vi "Merge Directories.vi"(6 "Ignore Read-Only? (FALSE)":bool, 8 "error in (no error)":errorcluster, 9 "Overwrite Existing Files? (FALSE)":bool, 10 "target directory path":path, 11 "source directory path":path) -> (0 "error out":errorcluster, 3 "dup target directory path":path)   [LabVIEW 2024]
doc: "Copies the contents of source directory into the destination directory. If source directory has subdirectories they will be copied into the destination directory recursively. Optionally, existing files may be overwritten, by setting the \"Overwrite Existing Files?\" input to TRUE. If you attempt to overwrite an existing file without setting to TRUE ans error will be returned. If FALSE, existing files will not be overwritten and no error wil be returned, Optionally, read-only files may be overwritten, by setting the \"Ignore Read-Only?\" input to TRUE. If you attempt to overwrite a read-only files without setting to TRUE an error will be returned. Optionally, by setting the \"Delete Source?\" input to TRUE the source directory will be deleted upon merge completion if no errors occured."
uses:
  <userlib>/_OpenG.lib/file/file.llb/Build Path - File Names Array__ogtk.vi
  <userlib>/_OpenG.lib/file/file.llb/Compare Two Paths - Scalar__ogtk.vi
  <userlib>/_OpenG.lib/file/file.llb/Build Path - Traditional - path__ogtk.vi
  <userlib>/_OpenG.lib/file/file.llb/Strip Path - Traditional__ogtk.vi
  <userlib>/_OpenG.lib/file/file.llb/openg_file.lvlib
  <userlib>/_OpenG.lib/error/error.llb/openg_error.lvlib
panel:
  # "OpenG Library.vi\n\nMerge Directories.vi\n\nCopies the contents of source directory into the destination directory.\n\nPlease visit http://www.OpenG.org to learn about the\nOpen Source LabVIEW software movement.\n\nNOTICE -- YOU MUST LEAVE THIS NOTICE IN PLACE.  PER THE TERMS OF THE LICENSE BELOW, YOU MAY SUBLICENSE THIS SOFTWARE \nIN ANY WAY THAT DOES NOT CONFLICT WITH THIS LICENSE.\n\n### BSD License (http://www.opensource.org/licenses/bsd-license.php) Begin ###\n \nCopyright (c) 2002-2004, Jim Kring <jim@jimkring.com>\nCopyright (c) 2002, Cal-Bay Systems, Inc. <info@calbay.com>\n\nAll rights reserved.\n\nRedistribution and use in source and binary forms, with or without modification, are permitted provided that the following conditions are met:\n\n    * Redistributions of source code must retain the above copyright notice, this list of conditions and the following disclaimer.\n    * Redistributions in binary form must reproduce the above copyright notice, this list of conditions and the following disclaimer in the \n       documentation and/or other materials provided with the distribution.\n    * Neither the name of SciWare, James Kring, Inc., nor the names of its contributors may be used to endorse or promote products derived \n       from this software without specific prior written permission.\n\nTHIS SOFTWARE IS PROVIDED BY THE COPYRIGHT HOLDERS AND CONTRIBUTORS \"AS IS\" AND ANY EXPRESS OR IMPLIED WARRANTIES, \nINCLUDING, BUT NOT LIMITED TO, THE IMPLIED WARRANTIES OF MERCHANTABILITY AND FITNESS FOR A PARTICULAR PURPOSE ARE \nDISCLAIMED. IN NO EVENT SHALL THE COPYRIGHT OWNER OR CONTRIBUTORS BE LIABLE FOR ANY DIRECT, INDIRECT, INCIDENTAL,\n SPECIAL, EXEMPLARY, OR CONSEQUENTIAL DAMAGES (INCLUDING, BUT NOT LIMITED TO, PROCUREMENT OF SUBSTITUTE GOODS OR \nSERVICES; LOSS OF USE, DATA, OR PROFITS; OR BUSINESS INTERRUPTION) HOWEVER CAUSED AND ON ANY THEORY OF LIABILITY, \nWHETHER IN CONTRACT, STRICT LIABILITY, OR TORT (INCLUDING NEGLIGENCE OR OTHERWISE) ARISING IN ANY WAY OUT OF THE USE \nOF THIS SOFTWARE, EVEN IF ADVISED OF THE POSSIBILITY OF SUCH DAMAGE.\n\n### BSD License End ###"
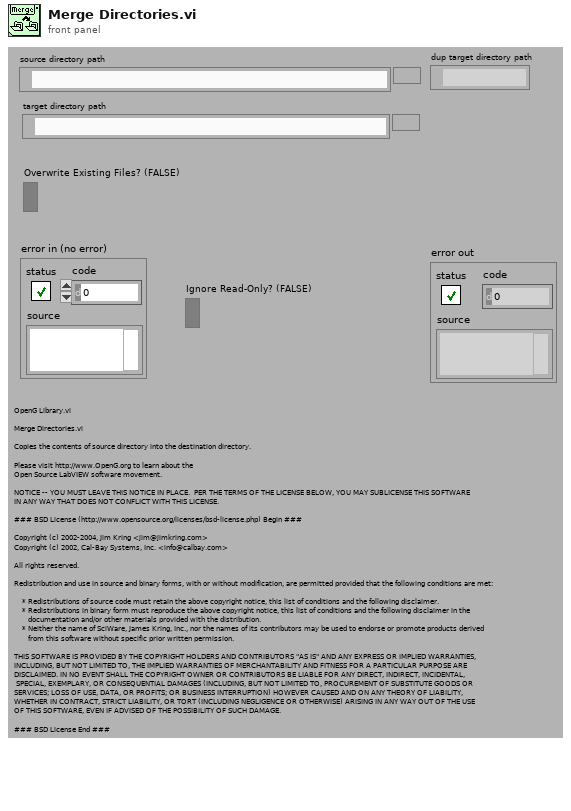
[diagram p1: front panel]
types:
  T1 = cluster{"Archive":bool, "Normal":bool, "Temporary":bool, "Compressed":bool, "Offline":bool, "Content Indexed":bool, "Encrypted (cannot set)":bool}
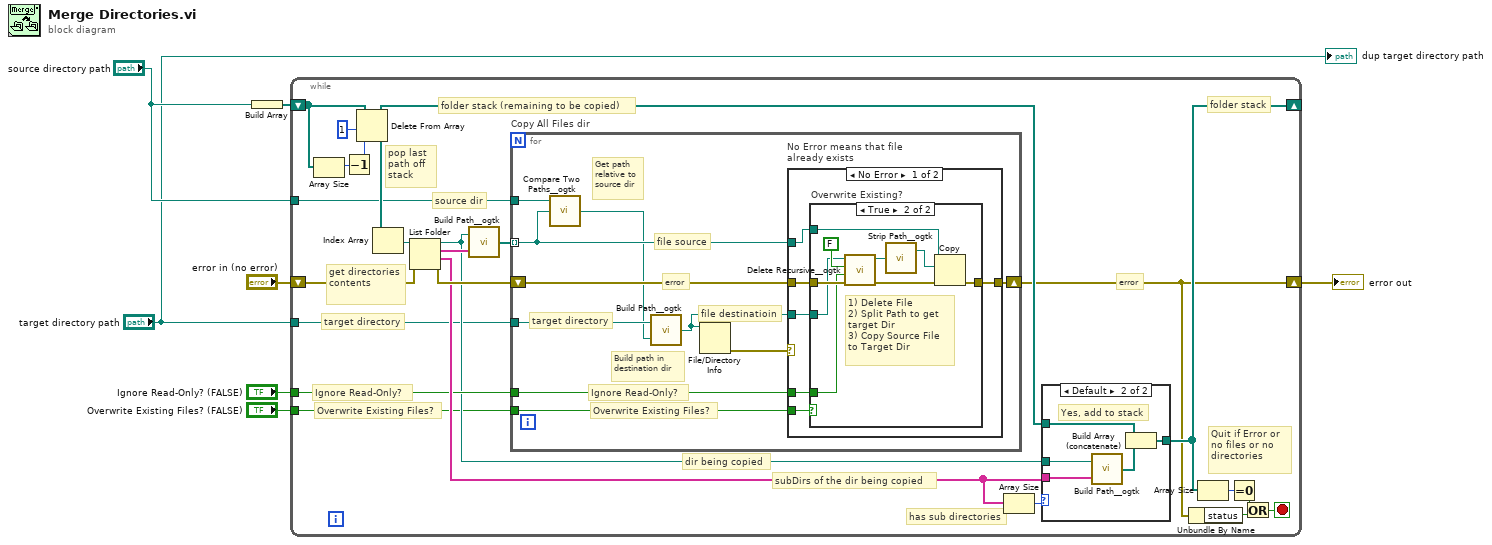
[diagram p0: block diagram]
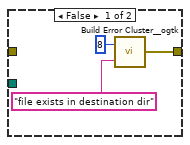
[diagram p3: hidden frame]
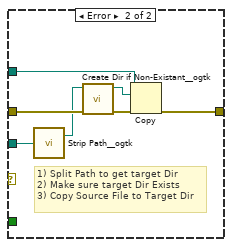
[diagram p4: hidden frame]
diagram:
  n1 = Build Array("source directory path") -> (w6:path[])
  n2 = while {
    shift-right: [w16] -> _
    shift-left: w6 -> [w19]
    shift-right: [w8] -> w3
    shift-left: "error in (no error)" -> [w20]
    tunnel: "Ignore Read-Only? (FALSE)" -> [w15]
    tunnel: "source directory path" -> [w11]
    tunnel: "target directory path" -> [w10]
    tunnel: "Overwrite Existing Files? (FALSE)" -> [w9]
    stop <- w21 stop-if-true
    (unwired) T1 {"Archive"=FALSE, "Normal"=FALSE, "Temporary"=FALSE, "Compressed"=FALSE, "Offline"=FALSE, "Content Indexed"=FALSE, "Encrypted (cannot set)"=FALSE} ("FileAttribute")
    # "folder stack"
    # "error"
    # "Overwrite Existing Files?"
    # "Ignore Read-Only?"
    # "target directory"
    # "subDirs of the dir being copied"
    # "dir being copied"
    # "folder stack (remaining to be copied)"
    # "source dir"
    # "get directories contents"
    # "pop last path off stack"
    # "Quit if Error or no files or no directories"
    # "has sub directories"
    n3 = Array Size(array=w19) -> (size(s)=w17:i32)
    n4 = Decrement(x=w17) -> (x-1=w18:i32)
    n5 = Delete From Array(array=w19, length=1 ("Length"), index=w18) -> (deleted portion=w30:path[], array with subset deleted=w25:path[])
    n6 = Index Array(array=w30) -> (element=w29:path)  [unwired: 1 in]
    n7 = List Folder(path=w29, error in=w20) -> (path out=w13:path, filenames=w14:string[], folder names=w26:string[], error out=w28:errorcluster)  [unwired: 2 in]
    n8 = call-poly <userlib>:"Build Path__ogtk.vi"("name or relative path"=w14, "base path"=w13) -> ("appended path"=w12:path[])
    n9 = for "Copy All Files dir" {
      shift-right: [w43] -> w8
      shift-left: w28 -> [w44]
      tunnel: w15 -> [w41]
      tunnel: w12 -> [w39] mode=indexing
      tunnel: w11 -> [w40]
      tunnel: w10 -> [w47]
      tunnel: w9 -> [w42]
      # "Ignore Read-Only?"
      # "Overwrite Existing Files?"
      # "file destinatioin"
      # "file source"
      # "target directory"
      # "error"
      # "Build path in destination dir"
      # "Get path relative to source dir"
      n10 = call-poly <userlib>:"Compare Two Paths__ogtk.vi"("path2"=w39, "path1"=w40) -> ("relative path from 1 to 2"=w38:path)  [unwired: 1 in, 2 out]
      n11 = call-poly <userlib>:"Build Path__ogtk.vi"("name or relative path"=w38, "base path"=w47) -> ("appended path"=w45:path)
      n12 = File/Directory Info(path=w45) -> (error out=w46:errorcluster)  [unwired: 1 in, 6 out]
      n13 = case "No Error means that file\nalready exists" shown="No Error" w46 {
        tunnel: w45 -> [w50 w70]
        tunnel: w39 -> [w49 w72]
        tunnel: w44 -> [w52 w69]
        tunnel: [w51 w71] -> w43
        tunnel: w42 -> [w53 _]
        tunnel: w41 -> [w48 _]
        frame No Error {
          n14 = case "Overwrite Existing?" shown="True" w53 {
            tunnel: w52 -> [_ w65]
            tunnel: [w54 w63] -> w51
            tunnel: w50 -> [_ w59]
            tunnel: w49 -> [_ w62]
            tunnel: w48 -> [_ w61]
            frame False {
              n15 = call <userlib>:"Build Error Cluster__ogtk.vi"("String to Prepend to source (\"\")"="file exists in destination dir" ("String to Prepend to source (\"\")"), "code"=8) -> ("error out"=w54:errorcluster)
            }
            frame True {
              # "1) Delete File\n2) Split Path to get target Dir\n3) Copy Source File to Target Dir"
              n16 = call <userlib>:"Delete Recursive__ogtk.vi"("error in (no error)"=w65, "Ignore Read-Only? (FALSE)"=w61, "Recursive? (FALSE)"=FALSE, "Path"=w59) -> ("error out"=w64:errorcluster, "dup Path"=w58:path)  [unwired: 6 in]
              n17 = call-poly <userlib>:"Strip Path__ogtk.vi"("path"=w58) -> ("stripped path"=w57:path)  [unwired: 1 out]
              n18 = Copy(8:w64, 10:w57, 11:w62) -> (0:w63:errorcluster)  [unwired: 2 in, 2 out]
            }
          }
        }
        frame Error {
          # "1) Split Path to get target Dir\n2) Make sure target Dir Exists\n3) Copy Source File to Target Dir"
          n19 = call-poly <userlib>:"Strip Path__ogtk.vi"("path"=w70) -> ("stripped path"=w66:path)  [unwired: 1 out]
          n20 = call <userlib>:"Create Dir if Non-Existant__ogtk.vi"("error in (no error)"=w69, "Directory Path"=w66) -> ("error out"=w68:errorcluster, "dup Directory Path"=w67:path)  [unwired: 7 in, 1 out]
          n21 = Copy(8:w68, 10:w67, 11:w72) -> (0:w71:errorcluster)  [unwired: 2 in, 2 out]
        }
      }
    }
    n22 = Array Size(array=w26) -> (size(s)=w27:i32)
    n23 = case shown="Default" w27 {
      tunnel: w13 -> [_ w33]
      tunnel: w26 -> [_ w37]
      tunnel: w25 -> [w32 w35]
      tunnel: [w32 w34] -> w16
      frame 0 {
      }
      frame Default {
        # "Yes, add to stack"
        n24 = call-poly <userlib>:"Build Path__ogtk.vi"("name or relative path"=w37, "base path"=w33) -> ("appended path"=w36:path[])
        n25 = Build Array (concatenate)(w35, w36) -> (w34:path[])
      }
    }
    n26 = Unbundle By Name(w8) -> ("status"=w23:bool)
    n27 = Array Size(array=w16) -> (size(s)=w24:i32)
    n28 = Equal To 0?(x=w24) -> (x = 0?=w22:bool)
    n29 = Or(x=w22, y=w23) -> (x .or. y?=w21:bool)
  }
  "error out" <- w3
  "dup target directory path" <- "target directory path"
